vi "Semantic_Dialogue_Array_Msg.vi"(8 "error in (no error)":errorcluster caption="错误输入（无错误）", 10 "值(信号)":T1, 11 "States.lvlib:Voice.lvclass":refnum<class "Voice.lvclass">) -> (0 "error out":errorcluster caption="错误输出", 3 "Process State out":refnum<class "State Actor.lvclass">)   [LabVIEW 2014, in "States.lvlib" / "Voice.lvclass"]
uses:
  Voice.lvclass
  ctl/Semantic_Voice_Array.ctl
  <vilib>/NI/Actors/State Actor/State Actor/State Actor.lvclass
  <vilib>/ActorFramework/Message Enqueuer/Message Enqueuer.lvclass/Message Enqueuer.ctl
  <vilib>/ActorFramework/Message Enqueuer/Enqueue.vi
  Global_var/Global_var.vi
  <vilib>/ActorFramework/Message Priority Queue/Priority Enqueue.vi
  ctl/Point.ctl
  Dialogue_lib/DialogueActor/Dialogue.lvclass
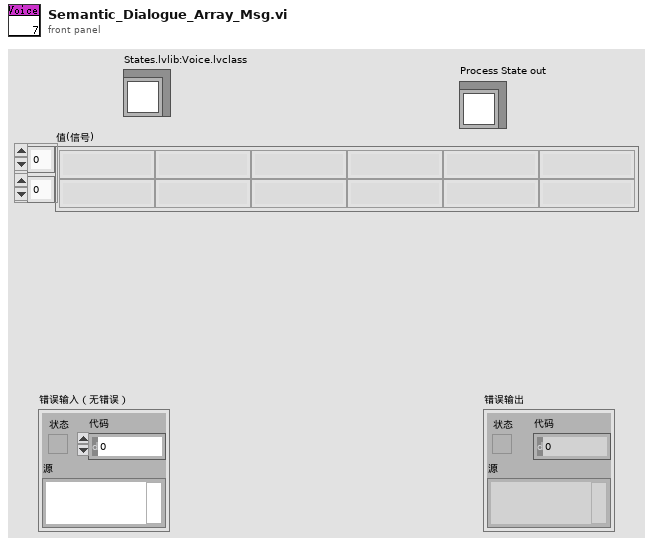
[diagram p1: front panel]
types:
  T1 = typedef "Semantic_Voice_Array.ctl" = string[][]
  T2 = cluster{"rot_z_max":dbl, "lin_x_max":dbl, "rot_z_min":dbl, "lin_x_min":dbl}
  T3 = typedef "Point.ctl" = cluster{"x":dbl, "y":dbl, "z":dbl}
  T4 = cluster{"now_pose_X":dbl, "now_pose_Y":dbl, "now_pose_Rot_deg":dbl}
  T5 = cluster{"起点":string, "终点":string, "动作":string, "方向":string, "距离":string, "速度":string}[]
  T6 = cluster{"起点":string, "终点":string, "动作":string, "方向":string, "距离":string, "速度":string}
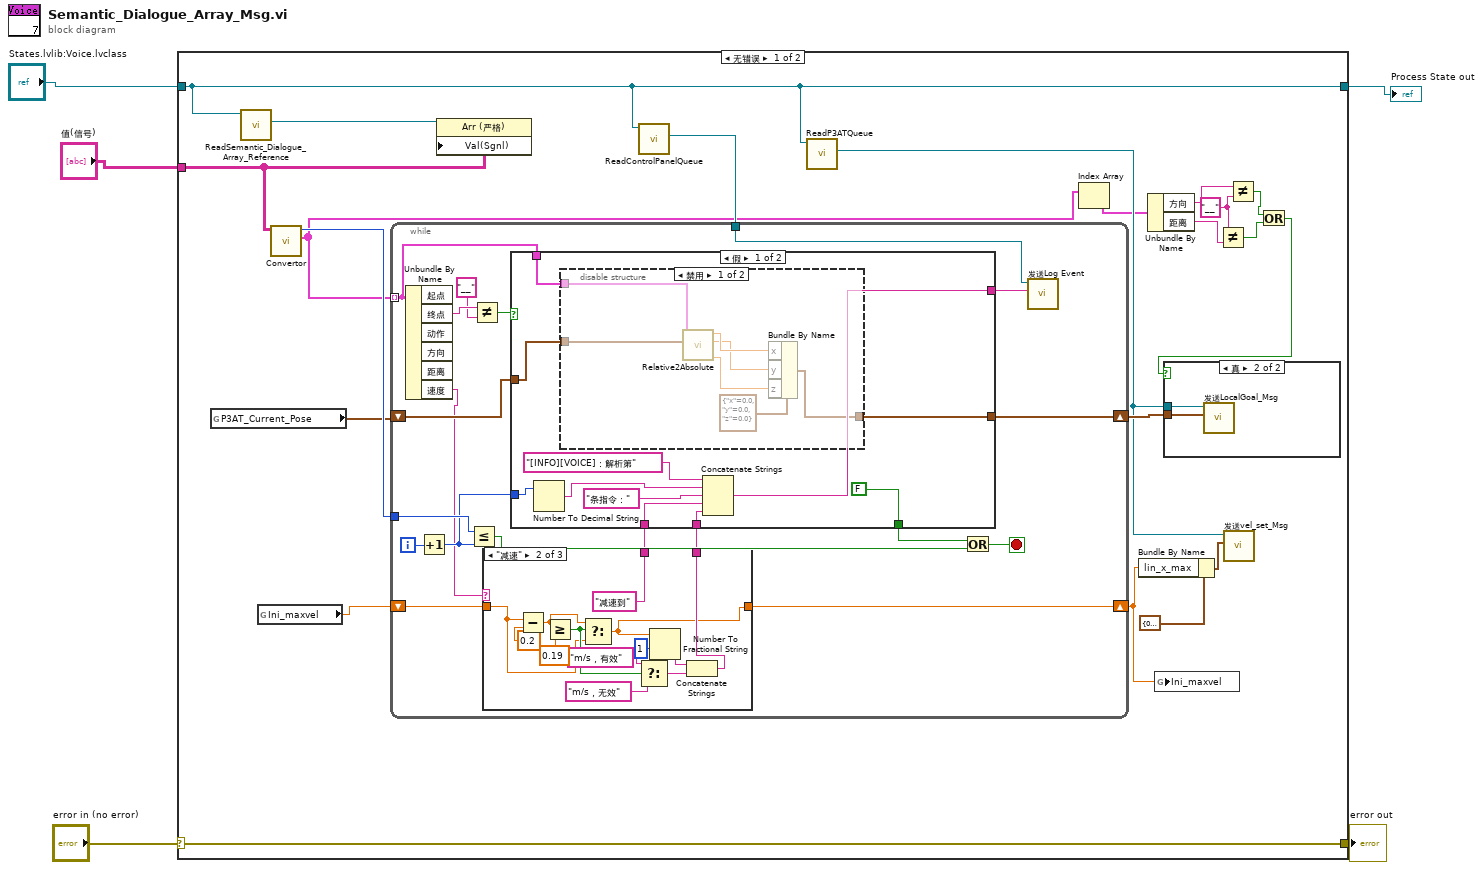
[diagram p0: block diagram]
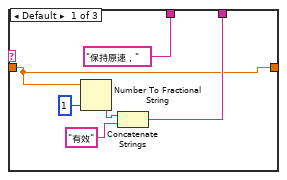
[diagram p3: hidden frame]
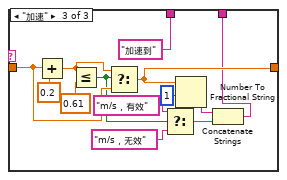
[diagram p4: hidden frame]
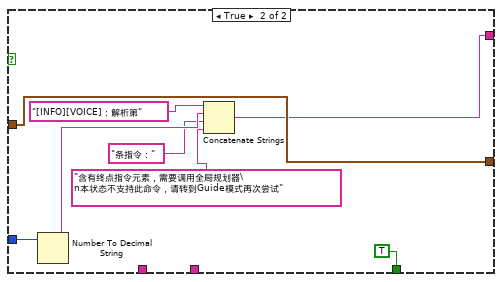
[diagram p6: hidden frame]
diagram:
  n1 = case shown="无错误" "error in (no error)" {
    selector: "error in (no error)" -> [w26 w106]
    tunnel: [w26 w106] -> w4
    tunnel: [w20 w107] -> w2
    tunnel: "States.lvlib:Voice.lvclass" -> [w20 w107]
    tunnel: "值(信号)" -> [w24 _]
    frame No Error {
      w10 = "__"
      n2 = global read "Global_var.vi" "P3AT_Current_Pose"() -> (w6:T4)
      n3 = call-dynamic "ReadSemantic_Dialogue_Array_Reference.vi"("CoordinatorState输入"=w20) -> ("Semantic_Dialogue_Array_Reference"=w25:refnum<vi>)  [unwired: 8 in, 2 out]
      n4 = global read "Global_var.vi" "Ini_maxvel"() -> (w22:dbl)
      n5 = call "Convertor.vi"("格式化机器人指令"=w24) -> ("机器人语音指令数据簇数组(Voice)"=w14:T5, "命令个数"=w23:i32)  [unwired: 8 in, 1 out]
      n6 = property class="Arr (严格)"(reference=w25, "Val(Sgnl)"=w24) -> ()  [unwired: 1 in, 2 out]
      n7 = call-dynamic "ReadControlPanelQueue.vi"("CoordinatorState输入"=w20) -> ("操作者框架:消息待入队列"=w19:refnum<class "Message Enqueuer.lvclass">)  [unwired: 8 in, 2 out]
      n8 = while {
        tunnel: w14 -> [w44] mode=indexing
        shift-right: [w42] -> w21
        shift-left: w6 -> [w41]
        tunnel: w23 -> [w39]
        shift-right: [w32] -> w18
        shift-left: w22 -> [w34]
        tunnel: w19 -> [w29]
        i -> [w43]
        stop <- w40 stop-if-true
        n9 = Unbundle By Name(w44) -> ("终点"=w47:string, "速度"=w35:string)  [unwired: 4 out]
        n10 = Increment(x=w43) -> (x+1=w38:i32)
        n11 = Less Or Equal?(x=w39, y=w38) -> (x <= y?=w37:bool)
        n12 = Not Equal?(x=w47, y="__") -> (x != y?=w45:bool)
        n13 = case shown="\"减速\"" w35 {
          tunnel: w34 -> [w49 w55 w75]
          tunnel: ["保持原速，" ("Event Text") "减速到" ("Event Text") "加速到" ("Event Text")] -> w33
          tunnel: [w49 w56 w70] -> w32
          tunnel: [w50 w57 w69] -> w31
          frame Default {
            n14 = Number To Fractional String(number=w49, precision (6)=i16 1 ("精度(6)")) -> (F-format string=w52:string)  [unwired: 2 in]
            n15 = Concatenate Strings(w52, "有效" ("Event Text")) -> (w50:string)
          }
          frame "减速" {
            n16 = Subtract(x=w55, y=0.2) -> (x-y=w64:dbl)
            n17 = Greater Or Equal?(x=w64, y=0.19) -> (x >= y?=w63:bool)
            n18 = Select(t=w64, s=w63, f=w55) -> (s? t:f=w56:dbl)
            n19 = Select(t="m/s，有效" ("Event Text"), s=w63, f="m/s，无效" ("Event Text")) -> (s? t:f=w60:string)
            n20 = Number To Fractional String(number=w56, precision (6)=i16 1 ("精度(6)")) -> (F-format string=w59:string)  [unwired: 2 in]
            n21 = Concatenate Strings(w59, w60) -> (w57:string)
          }
          frame "加速" {
            n22 = Add(x=w75, y=0.2) -> (x+y=w76:dbl)
            n23 = Less Or Equal?(x=w76, y=0.61) -> (x <= y?=w68:bool)
            n24 = Select(t=w76, s=w68, f=w75) -> (s? t:f=w70:dbl)
            n25 = Select(t="m/s，有效" ("Event Text"), s=w68, f="m/s，无效" ("Event Text")) -> (s? t:f=w72:string)
            n26 = Number To Fractional String(number=w70, precision (6)=i16 1 ("精度(6)")) -> (F-format string=w71:string)  [unwired: 2 in]
            n27 = Concatenate Strings(w71, w72) -> (w69:string)
          }
        }
        n28 = case shown="假" w45 {
          tunnel: [FALSE TRUE] -> w36
          tunnel: w44 -> [w88 _]
          tunnel: [w90 w99] -> w42
          tunnel: w41 -> [w89 w99]
          tunnel: w38 -> [w84 w104]
          tunnel: w33 -> [w82 _]
          tunnel: w31 -> [w81 _]
          tunnel: [w80 w98] -> w30
          frame False {
            n29 = Number To Decimal String(number=w84) -> (decimal integer string=w86:string)  [unwired: 1 in]
            n30 = disable-structure shown="禁用" {
              disable-tunnel: [w93 _] -> w90
              disable-tunnel: w89 -> [w92 _]
              disable-tunnel: w88 -> [w91 _]
              frame Disabled {
                n31 = call "Relative2Absolute.vi"("Ini_Pose"=w92, "机器人语音指令数据簇"=w91) -> ("Rot_deg"=w94:dbl, "y"=w95:dbl, "x"=w96:dbl)  [unwired: 7 in]
                n32 = Bundle By Name(cluster=T3 {"x"=0.0, "y"=0.0, "z"=0.0} ("值(信号)"), "x"=w96, "y"=w95, "z"=w94) -> (w93:T3)
              }
              frame Enabled {
              }
            }
            n33 = Concatenate Strings("[INFO][VOICE]：解析第" ("Event Text"), w86, "条指令：" ("Event Text"), w82, w81) -> (w80:string)
          }
          frame True {
            n34 = Number To Decimal String(number=w104) -> (decimal integer string=w102:string)  [unwired: 1 in]
            n35 = Concatenate Strings("[INFO][VOICE]：解析第" ("Event Text"), w102, "条指令：" ("Event Text"), "含有终点指令元素，需要调用全局规划器\n本状态不支持此命令，请转到Guide模式再次尝试" ("Event Text")) -> (w98:string)
          }
        }
        n36 = Or(x=w36, y=w37) -> (x .or. y?=w40:bool)
        n37 = call "发送Log Event.vi"("Event Text"=w30, "消息待入队列"=w29) -> ()  [unwired: 8 in, 2 out]
      }
      n38 = call-dynamic "ReadP3ATQueue.vi"("CoordinatorState输入"=w20) -> ("操作者框架:消息待入队列"=w15:refnum<class "Message Enqueuer.lvclass">)  [unwired: 8 in, 2 out]
      n39 = Index Array(array=w14) -> (element=w13:T6)  [unwired: 1 in]
      n40 = Bundle By Name(cluster=T2 {"rot_z_max"=0.0, "lin_x_max"=0.0, "rot_z_min"=0.0, "lin_x_min"=0.0} ("vel_set"), "lin_x_max"=w18) -> (w16:T2)
      n41 = Unbundle By Name(w13) -> ("方向"=w12:string, "距离"=w11:string)
      n42 = global write "Global_var.vi" "Ini_maxvel"(w18) -> ()
      n43 = Not Equal?(x=w10, y=w11) -> (x != y?=w8:bool)
      n44 = call "发送vel_set_Msg.vi"("值(信号)"=w16, "消息待入队列"=w15) -> ()  [unwired: 8 in, 2 out]
      n45 = Not Equal?(x=w12, y=w10) -> (x != y?=w9:bool)
      n46 = Or(x=w9, y=w8) -> (x .or. y?=w7:bool)
      n47 = case shown="真" w7 {
        tunnel: w21 -> [_ w28]
        tunnel: w15 -> [_ w27]
        frame False {
        }
        frame True {
          n48 = call "发送LocalGoal_Msg.vi"("值(信号)"=w28, "消息待入队列"=w27) -> ()  [unwired: 8 in, 2 out]
        }
      }
    }
    frame Error {
    }
  }
  "error out" <- w4
  "Process State out" <- w2
